vi "Main_18B.vi"() -> ()   [LabVIEW 2024]
uses:
  Utility/Universal Utility/TypeDefs_Utility/Cluster_Row-Column.ctl
  Utility/Universal Utility/TypeDefs_Utility/ENUM_4 Directions U-D-L-R.ctl
  6e548907-4bb0-43d1-b18c-1aae21799752.vi
  855a1de3-eed7-40d2-97cd-9cf78db46282.vi
  <vilib>/Utility/error.llb/Trim Whitespace.vi
  <vilib>/Utility/error.llb/Trim Whitespace One-Sided.vi
panel:
  out "Answer":T1
  out "Started":cluster{"Steps":u64, "Position":T1}[](array[cluster])
  out "sorted array":cluster{"Steps":u64, "Position":T1}[](array[cluster])
  out "Grid":string[][](array[string])
  in  "Puzzle Grid":T1={"R"=70, "C"=70}
  in  "Example Grid":T1={"R"=6, "C"=6}
  in  "Use Puzzle":bool
  out "Steps":u64
  in  "Puzzle":string="60,61\n19,47\n15,43\n15,48\n61,59\n23,51\n29,59\n10,25\n15,50\n26,39\n45,33\n7,29\n57,57\n11,25\n17,38\n3,1\n43,66\n57,55\n19,67\n2,47\n55,49\n13,25\n56,43\n9,2\n7,51\n23,61\n52,65\n11,47\n53,65\n21,47\n3,36\n11,38\n2,3\n1,27\n65,67\n64,63\n39,61\n23,52\n29,67\n69,31\n8,5\n16,69\n9,25\n61,63\n55,53\n7,50\n3,9\n2,41\n12,63\n28,57\n60,65\n55,34\n23,43\n51,68\n68,33\n53,43\n9,52\n21,1\n65,48\n6,27\n57,56\n65,39\n68,69\n67,38\n19,37\n19,63\n16,35\n38,61\n56,39\n24,47\n7,49\n65,59\n11,2\n10,61\n17,64\n60,57\n21,45\n67,59\n65,62\n14,59\n35,65\n37,53\n59,54\n3,19\n59,59\n24,49\n65,35\n5,20\n63,52\n1,51\n7,14\n68,67\n13,65\n8,37\n27,46\n1,12\n28,61\n21,61\n61,54\n41,67\n7,21\n61,58\n69,32\n69,57\n5,33\n1,10\n7,43\n45,57\n25,36\n14,53\n9,43\n27,39\n47,54\n67,41\n9,27\n55,61\n57,63\n65,46\n39,64\n9,33\n63,65\n25,62\n17,48\n8,57\n69,63\n49,35\n47,60\n7,25\n7,41\n59,43\n37,70\n5,28\n18,65\n62,33\n47,67\n19,61\n67,60\n25,44\n69,41\n11,49\n5,37\n12,31\n51,53\n33,63\n23,47\n29,37\n69,55\n23,7\n39,59\n1,0\n39,66\n18,37\n51,57\n10,41\n3,49\n23,39\n59,42\n45,58\n23,56\n67,69\n44,65\n64,69\n4,19\n2,51\n11,43\n1,48\n45,61\n1,29\n32,63\n7,53\n13,27\n52,61\n11,23\n9,63\n5,6\n1,14\n40,69\n19,43\n29,39\n43,69\n53,55\n3,7\n19,62\n27,43\n59,39\n63,57\n41,68\n7,20\n16,45\n26,37\n22,59\n13,47\n13,50\n39,50\n19,29\n51,60\n17,30\n8,61\n9,49\n42,65\n3,31\n56,37\n15,41\n2,31\n5,15\n19,41\n61,32\n1,25\n1,4\n59,67\n6,41\n15,67\n3,35\n61,36\n31,59\n19,3\n65,55\n65,60\n61,55\n57,68\n56,49\n1,19\n3,11\n66,41\n1,15\n66,69\n9,41\n63,39\n2,15\n13,8\n55,32\n19,57\n49,55\n69,40\n67,67\n10,57\n19,51\n2,7\n22,29\n24,41\n5,4\n61,45\n59,63\n11,32\n60,39\n57,35\n24,43\n65,53\n26,69\n21,65\n6,17\n11,34\n67,55\n26,45\n69,43\n30,61\n7,22\n27,47\n7,37\n58,65\n12,41\n9,39\n35,69\n46,63\n13,67\n67,35\n39,69\n15,26\n63,37\n13,45\n43,67\n17,43\n14,61\n57,69\n21,40\n21,56\n69,44\n41,51\n67,43\n37,67\n59,64\n35,59\n0,33\n1,41\n69,56\n31,63\n31,52\n18,57\n13,23\n8,31\n56,53\n7,19\n9,40\n69,66\n9,23\n11,37\n5,29\n22,63\n25,57\n11,46\n1,3\n6,35\n3,2\n8,9\n69,59\n67,49\n53,67\n3,53\n46,67\n49,61\n27,61\n1,33\n54,59\n10,23\n23,41\n6,51\n29,40\n1,37\n14,25\n20,69\n4,35\n15,38\n8,23\n5,19\n23,53\n58,43\n34,63\n63,41\n65,56\n14,43\n21,49\n28,69\n23,57\n57,41\n22,19\n62,35\n11,50\n1,13\n9,20\n28,67\n61,67\n20,43\n58,35\n13,24\n8,53\n3,50\n27,41\n40,67\n0,37\n10,29\n57,39\n31,65\n15,39\n66,51\n10,1\n12,5\n7,44\n3,15\n11,35\n23,38\n58,53\n19,49\n10,65\n39,67\n57,60\n18,67\n33,69\n1,20\n42,63\n37,63\n13,35\n63,55\n11,15\n61,53\n68,59\n51,65\n1,49\n9,46\n19,59\n67,39\n3,45\n50,65\n53,51\n47,61\n65,50\n7,28\n8,35\n21,57\n63,61\n11,33\n3,21\n15,64\n10,15\n25,69\n51,59\n53,39\n7,35\n69,35\n5,10\n3,5\n47,47\n43,65\n37,69\n61,33\n49,56\n25,43\n59,32\n54,55\n51,43\n62,47\n27,69\n10,9\n35,56\n48,67\n57,43\n1,21\n25,41\n5,7\n17,65\n18,39\n61,65\n17,69\n19,45\n55,67\n1,31\n31,57\n17,41\n1,43\n63,43\n44,63\n11,45\n54,69\n55,58\n58,39\n11,36\n4,51\n1,6\n52,67\n16,59\n23,70\n65,61\n59,57\n27,37\n3,16\n56,67\n7,30\n3,47\n3,18\n29,38\n59,36\n69,69\n49,59\n4,25\n43,59\n63,59\n17,47\n0,23\n11,24\n1,1\n37,58\n47,64\n5,48\n5,53\n22,69\n11,29\n61,57\n30,59\n20,59\n11,31\n3,29\n12,43\n15,44\n67,31\n15,36\n43,62\n57,61\n17,39\n67,45\n53,46\n9,3\n18,49\n13,61\n53,62\n66,45\n13,37\n39,65\n11,27\n25,45\n59,69\n21,46\n67,53\n55,70\n17,34\n51,44\n36,61\n63,64\n29,61\n67,37\n61,56\n64,39\n29,65\n42,69\n68,47\n29,36\n17,51\n65,63\n19,32\n69,37\n25,59\n65,33\n13,28\n61,51\n66,53\n38,65\n57,37\n3,38\n11,51\n52,57\n22,41\n65,41\n53,53\n33,56\n27,63\n35,61\n67,44\n69,61\n35,66\n23,45\n3,33\n14,29\n16,65\n61,70\n61,43\n43,57\n7,32\n14,37\n40,63\n61,42\n70,39\n63,40\n53,50\n24,51\n21,39\n2,11\n51,66\n15,62\n62,51\n17,33\n17,29\n51,61\n8,27\n5,45\n53,56\n13,2\n59,52\n61,49\n68,53\n9,51\n58,57\n4,13\n35,63\n21,69\n51,69\n30,63\n12,39\n48,59\n37,68\n45,63\n59,41\n62,67\n5,21\n3,44\n7,42\n19,65\n65,32\n7,17\n64,43\n6,47\n27,60\n1,45\n49,65\n26,63\n1,22\n8,39\n54,33\n7,3\n54,49\n29,63\n65,51\n54,39\n3,37\n9,21\n4,33\n66,57\n7,15\n6,37\n17,46\n58,59\n52,49\n21,37\n1,23\n52,41\n55,64\n3,23\n69,62\n20,41\n2,29\n65,43\n17,67\n29,69\n31,61\n53,42\n51,55\n53,69\n57,67\n7,47\n51,58\n55,57\n63,63\n2,9\n24,59\n17,19\n57,65\n5,2\n0,45\n19,55\n7,23\n9,29\n61,44\n41,61\n25,5\n69,53\n5,47\n51,67\n65,65\n13,40\n2,35\n13,29\n67,48\n9,34\n4,47\n9,53\n21,34\n66,65\n11,41\n2,17\n67,54\n17,59\n11,53\n17,52\n5,25\n4,53\n29,47\n32,61\n15,63\n48,49\n64,55\n25,39\n11,68\n13,64\n65,36\n19,69\n25,48\n24,65\n31,47\n59,65\n55,69\n10,51\n13,46\n27,64\n51,35\n22,49\n69,45\n27,67\n49,68\n65,69\n25,66\n34,61\n68,35\n12,27\n1,39\n59,38\n69,49\n53,61\n49,69\n9,31\n26,59\n51,32\n4,31\n24,57\n64,65\n70,31\n49,57\n63,66\n23,37\n56,41\n35,58\n67,65\n5,35\n57,33\n22,61\n69,46\n17,31\n11,14\n35,64\n64,33\n57,53\n54,61\n37,45\n53,49\n5,39\n8,13\n67,40\n24,37\n67,66\n27,65\n10,43\n0,51\n17,60\n13,31\n7,2\n12,65\n55,59\n33,57\n67,63\n49,46\n21,43\n65,37\n57,59\n21,53\n15,47\n19,36\n59,35\n5,5\n5,31\n61,35\n14,67\n45,68\n6,25\n3,22\n2,43\n50,51\n9,45\n3,26\n20,65\n2,39\n20,47\n61,64\n59,61\n1,42\n3,41\n19,31\n56,57\n43,60\n63,58\n37,65\n58,33\n55,41\n65,49\n53,57\n43,50\n11,48\n5,40\n13,59\n9,57\n26,57\n60,67\n63,67\n6,3\n19,53\n69,67\n59,60\n17,37\n11,26\n28,63\n53,45\n17,27\n17,62\n59,37\n3,28\n49,63\n53,33\n56,61\n6,33\n18,59\n59,68\n41,69\n19,54\n31,37\n62,39\n7,52\n21,52\n27,59\n41,65\n7,7\n11,39\n62,69\n9,47\n16,41\n60,31\n9,59\n11,30\n1,9\n7,1\n21,66\n64,37\n65,57\n69,47\n39,57\n25,47\n5,9\n7,33\n1,17\n69,51\n61,41\n11,16\n6,19\n36,63\n38,57\n55,55\n1,28\n47,69\n4,5\n59,33\n63,35\n62,49\n49,67\n37,61\n5,38\n18,43\n7,0\n54,67\n25,37\n11,66\n67,62\n16,51\n63,69\n5,8\n61,39\n15,29\n68,51\n0,7\n69,64\n21,59\n43,63\n11,7\n63,33\n21,51\n1,26\n49,53\n10,35\n57,34\n70,55\n22,43\n61,38\n3,3\n21,50\n5,27\n23,67\n4,41\n3,17\n20,61\n63,48\n67,51\n66,33\n39,62\n20,53\n68,49\n54,43\n27,5\n25,63\n20,21\n39,63\n55,43\n13,49\n5,23\n8,49\n65,42\n8,25\n4,23\n27,52\n20,37\n53,41\n66,37\n3,25\n18,45\n22,55\n48,65\n9,11\n3,39\n14,31\n65,68\n36,67\n15,66\n55,54\n42,45\n61,69\n3,46\n8,47\n64,53\n69,39\n51,48\n3,13\n2,33\n19,39\n3,27\n33,59\n23,65\n15,30\n23,68\n65,31\n53,59\n55,36\n9,37\n22,25\n19,42\n23,69\n14,49\n17,40\n69,36\n47,65\n55,35\n39,60\n22,37\n60,51\n21,67\n12,47\n9,35\n55,33\n69,65\n68,57\n28,39\n62,55\n57,40\n1,5\n5,44\n65,47\n11,63\n5,1\n54,51\n21,44\n25,61\n61,37\n9,54\n22,65\n25,65\n17,45\n67,42\n67,47\n25,67\n57,66\n23,59\n61,47\n45,66\n62,61\n13,43\n7,16\n45,65\n64,59\n20,31\n17,61\n7,39\n41,63\n27,66\n1,47\n15,65\n21,55\n15,20\n55,52\n18,51\n24,61\n13,41\n62,43\n55,65\n25,68\n67,33\n51,63\n50,43\n23,46\n4,11\n56,63\n5,51\n11,67\n20,57\n5,30\n63,51\n3,24\n14,41\n59,55\n23,49\n15,45\n8,43\n32,65\n66,35\n63,53\n69,60\n15,61\n67,57\n11,13\n61,61\n14,45\n69,42\n25,40\n1,35\n69,33\n63,47\n49,70\n1,11\n61,62\n29,57\n13,63\n33,61\n9,55\n9,58\n62,59\n19,68\n15,49\n69,52\n48,63\n47,56\n17,63\n17,68\n5,49\n20,49\n51,49\n35,9\n5,63\n27,1\n37,39\n37,16\n51,4\n37,8\n63,8\n49,31\n33,13\n59,21\n55,7\n60,49\n36,23\n17,21\n59,17\n19,33\n29,12\n39,35\n13,4\n9,19\n61,7\n45,36\n31,53\n69,0\n25,18\n50,1\n53,15\n60,11\n38,3\n43,25\n13,57\n34,23\n32,23\n63,45\n19,9\n12,61\n39,7\n43,15\n9,13\n47,29\n45,59\n1,7\n47,70\n57,27\n15,56\n37,28\n7,57\n57,10\n40,37\n33,53\n24,5\n25,1\n37,11\n13,14\n51,29\n39,19\n43,17\n49,43\n32,5\n27,19\n35,31\n44,15\n11,9\n49,3\n30,7\n36,27\n41,15\n66,27\n21,9\n43,23\n27,4\n49,39\n39,5\n11,65\n23,9\n56,5\n47,49\n33,28\n48,25\n43,53\n15,53\n48,3\n48,11\n47,2\n29,19\n5,41\n45,30\n49,7\n32,25\n31,69\n65,15\n31,36\n29,17\n23,54\n25,35\n12,53\n69,4\n20,7\n33,27\n63,25\n42,37\n33,12\n53,3\n21,19\n61,21\n45,16\n41,13\n31,30\n53,23\n45,7\n5,55\n31,19\n51,37\n23,1\n27,2\n53,17\n39,51\n40,9\n69,12\n37,37\n13,21\n19,2\n16,3\n35,39\n48,43\n43,49\n29,35\n19,34\n51,19\n15,35\n11,6\n60,23\n21,29\n50,9\n53,11\n53,47\n39,25\n37,54\n28,49\n55,8\n49,19\n21,25\n42,57\n1,61\n1,64\n47,59\n1,65\n59,27\n59,29\n42,27\n55,37\n10,7\n44,1\n15,16\n57,19\n69,17\n54,35\n17,24\n43,51\n13,51\n34,43\n55,63\n69,19\n28,19\n27,21\n31,5\n26,7\n20,63\n51,41\n31,11\n51,45\n45,13\n27,7\n7,68\n23,27\n57,3\n57,25\n25,51\n8,17\n41,28\n32,57\n49,47\n37,34\n26,55\n45,43\n48,29\n51,39\n25,25\n3,57\n56,25\n39,27\n20,9\n27,31\n69,7\n54,47\n69,13\n52,15\n69,3\n62,19\n35,50\n16,17\n27,23\n63,14\n55,16\n61,11\n42,53\n66,5\n31,15\n3,43\n18,9\n17,20\n43,11\n23,21\n62,3\n52,21\n7,5\n33,7\n65,11\n39,46\n61,6\n37,49\n39,49\n31,9\n42,19\n47,33\n31,20\n58,13\n61,8\n24,33\n66,23\n51,40\n35,55\n45,53\n43,55\n35,5\n32,39\n47,21\n41,48\n55,19\n11,59\n45,27\n17,23\n27,24\n23,24\n25,3\n7,59\n35,48\n11,61\n1,62\n64,13\n46,57\n39,0\n6,63\n33,46\n31,13\n33,41\n37,2\n19,5\n48,53\n69,9\n5,54\n33,9\n57,22\n43,7\n15,51\n67,18\n39,44\n41,1\n6,59\n33,43\n57,13\n31,16\n55,5\n31,42\n15,17\n22,15\n42,21\n28,33\n7,66\n37,50\n15,9\n23,8\n21,0\n42,49\n16,27\n29,9\n67,5\n39,17\n11,12\n5,3\n19,18\n59,53\n47,39\n59,9\n45,21\n5,67\n13,11\n15,55\n1,66\n47,28\n49,11\n30,47\n35,32\n41,53\n27,30\n38,39\n44,37\n47,9\n5,13\n31,18\n11,10\n38,7\n37,9\n49,8\n39,31\n29,22\n25,14\n29,53\n12,9\n48,45\n27,55\n13,13\n28,27\n35,30\n38,33\n68,15\n33,37\n69,29\n55,51\n45,67\n65,23\n52,53\n51,25\n15,7\n25,53\n69,14\n44,5\n65,9\n13,15\n51,9\n65,27\n18,27\n51,1\n43,1\n47,7\n51,52\n41,21\n19,4\n23,2\n35,20\n44,55\n37,35\n11,57\n25,55\n40,19\n51,30\n51,5\n9,4\n47,16\n69,21\n25,21\n20,19\n12,59\n10,19\n13,36\n35,42\n43,8\n7,55\n44,45\n37,19\n50,63\n37,13\n55,45\n65,5\n56,7\n57,45\n54,63\n55,0\n35,2\n29,7\n17,13\n30,65\n15,19\n48,19\n7,9\n13,34\n37,1\n31,68\n59,1\n53,35\n41,22\n15,4\n56,23\n11,19\n41,17\n47,25\n19,10\n39,39\n65,1\n21,33\n15,23\n51,20\n40,57\n41,16\n6,69\n45,69\n46,51\n21,21\n45,52\n11,3\n41,57\n36,33\n45,48\n69,15\n67,12\n23,33\n22,13\n59,8\n43,45\n59,13\n29,5\n4,67\n39,55\n38,47\n27,15\n26,19\n70,23\n67,19\n42,55\n30,67\n25,23\n35,3\n25,29\n57,5\n6,55\n39,47\n33,31\n35,68\n47,5\n41,58\n33,65\n29,58\n28,55\n40,55\n67,23\n46,39\n53,13\n51,3\n47,63\n7,56\n43,40\n41,24\n30,5\n26,9\n37,21\n13,56\n31,33\n35,67\n15,33\n7,13\n21,27\n44,21\n46,7\n53,14\n33,55\n15,2\n43,41\n30,45\n59,23\n11,54\n25,19\n35,25\n42,43\n23,63\n37,10\n47,26\n61,1\n15,6\n59,5\n31,2\n21,15\n46,3\n19,35\n3,56\n3,55\n3,63\n47,34\n35,57\n51,31\n41,30\n5,58\n18,7\n32,31\n7,6\n41,5\n48,9\n3,51\n28,17\n33,17\n27,14\n47,27\n41,14\n49,23\n47,19\n24,9\n45,5\n55,9\n9,15\n24,29\n39,3\n39,30\n9,68\n63,10\n54,7\n59,45\n14,7\n36,37\n43,5\n45,18\n65,45\n59,25\n19,27\n67,7\n58,19\n36,11\n13,55\n35,41\n51,33\n33,44\n63,28\n29,41\n12,69\n32,47\n40,25\n46,47\n30,27\n53,19\n23,31\n41,41\n7,67\n68,11\n40,3\n1,63\n22,33\n68,21\n60,19\n7,45\n45,32\n11,5\n49,5\n45,9\n53,16\n65,19\n30,9\n67,29\n55,1\n31,21\n61,12\n63,19\n5,43\n32,41\n41,39\n16,21\n4,63\n62,45\n33,45\n14,17\n17,53\n17,32\n51,7\n56,15\n39,21\n53,2\n43,13\n33,39\n25,49\n50,17\n30,33\n56,27\n41,11\n25,33\n45,40\n47,23\n17,1\n55,15\n59,28\n54,11\n11,17\n57,48\n31,49\n41,55\n15,31\n23,5\n53,27\n35,17\n66,21\n23,19\n33,3\n33,35\n19,15\n69,26\n37,57\n13,22\n38,53\n57,4\n49,1\n41,37\n47,37\n50,37\n67,11\n67,13\n22,7\n29,43\n29,16\n35,29\n41,43\n67,61\n1,69\n30,19\n39,37\n47,43\n65,20\n67,21\n39,15\n51,17\n36,1\n43,31\n42,61\n50,33\n13,0\n21,6\n52,9\n11,1\n19,19\n63,0\n44,3\n26,33\n31,51\n36,25\n49,37\n63,7\n63,49\n39,26\n61,26\n45,45\n13,5\n53,38\n47,45\n18,3\n53,21\n53,31\n21,63\n31,25\n43,27\n15,37\n15,27\n59,24\n25,13\n47,57\n13,20\n13,53\n56,1\n15,25\n33,38\n26,23\n35,36\n43,35\n25,9\n41,3\n46,11\n31,28\n24,3\n25,15\n58,25\n37,48\n45,42\n29,54\n45,25\n17,14\n63,26\n22,27\n40,35\n29,33\n35,23\n38,15\n2,59\n68,27\n19,1\n38,41\n11,55\n23,25\n68,7\n33,40\n31,50\n50,23\n53,5\n2,53\n53,29\n50,49\n23,3\n53,24\n38,27\n65,17\n32,3\n37,31\n30,23\n31,3\n37,3\n19,23\n23,35\n46,5\n24,13\n43,42\n46,45\n34,17\n7,11\n27,57\n26,13\n53,18\n30,55\n69,6\n47,1\n69,1\n49,27\n7,61\n39,13\n39,24\n65,21\n15,5\n27,3\n21,7\n43,6\n59,15\n5,57\n41,32\n3,67\n27,35\n59,30\n45,35\n41,27\n64,21\n39,1\n61,15\n31,27\n14,69\n65,13\n38,5\n59,49\n63,5\n45,11\n60,45\n60,17\n52,35\n31,31\n27,6\n25,26\n51,21\n29,29\n51,38\n68,23\n28,21\n9,62\n47,20\n57,51\n68,19\n15,57\n33,29\n32,59\n1,53\n54,19\n25,20\n9,1\n58,51\n17,6\n37,29\n57,18\n33,68\n42,3\n55,11\n61,14\n56,31\n5,60\n44,27\n20,27\n64,5\n15,1\n37,41\n31,35\n31,45\n67,2\n26,29\n68,17\n42,39\n17,55\n13,33\n31,56\n25,22\n58,1\n37,59\n35,8\n32,53\n35,4\n68,29\n61,2\n48,13\n45,60\n55,21\n47,38\n55,2\n67,8\n17,49\n7,63\n63,1\n7,69\n65,30\n37,22\n51,22\n5,17\n17,11\n37,44\n35,47\n30,13\n33,1\n39,43\n35,16\n13,19\n49,15\n17,18\n36,21\n63,13\n55,29\n65,29\n39,33\n41,45\n34,59\n53,1\n50,7\n17,7\n17,54\n61,5\n21,22\n48,51\n41,25\n48,15\n33,34\n21,5\n46,31\n8,65\n41,4\n47,14\n43,61\n37,7\n1,57\n40,1\n34,51\n61,27\n24,25\n61,23\n17,17\n36,45\n33,67\n69,25\n57,1\n63,3\n14,13\n37,5\n49,49\n37,33\n60,3\n66,25\n29,27\n6,13\n21,31\n59,3\n47,55\n9,17\n34,13\n9,60\n1,68\n47,35\n45,29\n35,37\n60,21\n34,27\n63,21\n67,17\n49,58\n2,55\n63,31\n55,25\n23,6\n15,21\n28,5\n41,59\n43,29\n57,17\n47,13\n25,10\n63,9\n34,37\n52,27\n47,24\n49,29\n11,56\n31,55\n33,26\n53,30\n59,6\n5,61\n37,55\n37,36\n70,9\n42,15\n59,47\n20,25\n3,69\n30,35\n35,11\n59,51\n51,54\n26,1\n55,3\n11,69\n17,3\n51,11\n13,69\n20,29\n53,4\n63,29\n15,69\n67,9\n46,23\n49,22\n41,47\n15,13\n65,24\n9,61\n54,25\n27,49\n5,11\n49,0\n61,3\n15,22\n67,3\n37,17\n29,21\n37,18\n50,3\n28,41\n23,22\n42,1\n55,23\n55,39\n13,9\n21,12\n29,3\n31,39\n38,21\n39,38\n25,27\n66,15\n65,3\n37,51\n45,41\n62,5\n51,27\n27,50\n35,6\n23,11\n47,41\n41,9\n21,17\n45,1\n4,57\n63,11\n45,51\n48,41\n46,49\n35,35\n39,45\n27,53\n46,43\n63,30\n9,18\n28,9\n0,57\n5,62\n52,3\n23,55\n9,9\n51,24\n17,56\n53,63\n35,7\n3,70\n63,12\n2,65\n43,21\n50,27\n20,15\n36,17\n64,3\n57,12\n62,29\n41,31\n33,51\n59,31\n29,13\n37,43\n45,37\n57,31\n34,53\n28,11\n59,19\n49,51\n54,5\n45,44\n45,10\n43,37\n47,22\n9,67\n65,6\n29,0\n19,17\n32,7\n36,13\n57,11\n52,29\n44,23\n29,31\n27,27\n25,0\n69,11\n31,66\n33,47\n21,3\n35,43\n39,9\n49,18\n47,36\n61,17\n29,14\n59,11\n37,25\n29,48\n61,10\n66,3\n57,23\n25,16\n54,27\n15,3\n26,53\n27,13\n67,10\n41,7\n13,10\n50,35\n53,9\n29,49\n53,25\n60,15\n51,51\n70,17\n25,4\n29,25\n63,22\n37,30\n33,20\n37,56\n19,16\n50,55\n33,10\n61,19\n51,13\n58,15\n28,35\n32,33\n61,9\n29,11\n41,49\n31,17\n3,58\n51,12\n35,33\n50,41\n43,9\n35,19\n34,7\n17,9\n69,23\n35,45\n47,51\n31,44\n57,7\n68,3\n30,43\n33,23\n57,49\n41,35\n58,9\n51,23\n17,57\n51,10\n35,51\n38,19\n13,7\n40,39\n67,27\n61,25\n53,7\n40,49\n40,29\n45,34\n51,26\n31,1\n34,9\n3,62\n57,30\n15,15\n43,47\n42,9\n64,1\n13,3\n30,51\n33,19\n9,7\n41,52\n61,4\n40,53\n63,16\n49,21\n44,29\n55,27\n11,22\n34,19\n61,24\n15,32\n19,21\n7,64\n35,49\n13,39\n51,15\n50,13\n17,0\n18,21\n55,22\n45,23\n24,17\n31,7\n27,29\n48,61\n43,43\n57,29\n37,15\n37,47\n33,4\n37,52\n29,45\n31,29\n49,45\n7,8\n5,69\n41,23\n35,15\n38,35\n35,53\n28,43\n43,34\n15,59\n17,5\n31,23\n43,20\n63,24\n27,17\n65,16\n35,21\n47,6\n57,21\n61,29\n63,18\n32,17\n39,41\n23,13\n7,27\n44,51\n1,55\n33,5\n3,65\n7,65\n47,31\n54,21\n17,35\n27,33\n65,10\n53,10\n53,37\n49,9\n13,58\n48,31\n19,11\n45,8\n25,17\n63,23\n23,23\n33,25\n3,59\n10,13\n22,17\n25,54\n39,11\n33,33\n44,11\n22,11\n33,21\n45,26\n26,27\n34,1\n27,51\n52,37\n44,57\n63,15\n18,11\n46,27\n46,13\n26,49\n3,61\n29,32\n67,1\n47,15\n45,31\n12,17\n50,31\n59,7\n23,29\n28,45\n55,17\n27,45\n49,25\n24,31\n43,19\n16,57\n65,7\n19,7\n38,13\n34,31\n47,11\n69,27\n4,65\n42,11\n42,17\n32,51\n4,15\n45,49\n27,11\n25,32\n33,14\n9,69\n43,33\n39,29\n17,15\n65,25\n69,5\n47,17\n52,45\n11,11\n49,13\n57,9\n41,46\n58,47\n8,69\n13,52\n31,41\n45,39\n9,5\n41,29\n56,13\n43,32\n58,3\n46,19\n6,11\n30,29\n20,3\n45,3\n17,28\n18,25\n48,39\n60,47\n61,13\n19,25\n25,31\n22,31\n44,13\n29,23\n37,23\n38,11\n5,46\n40,17\n1,67\n21,13\n40,43\n49,41\n33,15\n27,25\n30,3\n21,23\n12,19\n45,19\n47,3\n34,35\n1,59\n58,21\n69,28\n48,35\n29,26\n63,17\n8,11\n67,30\n20,23\n54,45\n22,3\n43,39\n18,15\n24,35\n55,13\n33,11\n29,15\n23,15\n39,14\n56,45\n38,43\n15,12\n16,11\n35,40\n45,55\n52,19\n13,1\n51,47\n56,11\n44,47\n41,19\n5,59\n62,21\n29,8\n29,24\n41,12\n40,41\n31,67\n65,8\n47,53\n49,17\n39,8\n28,29\n25,11\n49,6\n45,54\n49,33\n25,7\n23,17\n45,17\n32,11\n45,47\n58,45\n65,18\n35,13\n29,51\n55,28\n35,46\n59,16\n34,25\n19,13\n13,17\n67,15\n1,60\n5,65\n27,9\n23,20\n43,3\n29,55\n42,31\n57,15\n17,12\n7,31\n41,6\n20,13\n39,53\n63,27\n53,6\n15,8\n33,49\n39,23\n21,11\n35,1\n61,31\n57,28\n55,47\n31,43\n35,54\n40,5\n26,11\n21,35\n43,24\n50,15\n36,41\n18,29\n45,15\n57,47\n11,21\n3,68\n17,25\n21,41\n37,27\n60,27\n67,25\n42,35\n9,65\n33,48\n33,70\n64,27\n56,19\n35,27\n15,11\n41,33\n55,31\n29,1\n30,16\n57,26\n52,16\n36,7\n41,2\n36,29\n6,22\n68,61\n27,16\n56,9\n60,54\n70,37\n66,49\n61,40\n12,55\n0,42\n44,41\n40,48\n64,52\n56,6\n12,8\n63,50\n26,28\n17,26\n47,12\n21,18\n66,48\n66,4\n52,22\n54,46\n47,42\n28,60\n60,41\n64,42\n40,51\n24,18\n0,59\n63,2\n3,32\n31,64\n6,24\n58,48\n42,60\n60,33\n42,8\n5,24\n46,69\n48,37\n58,64\n24,24\n20,39\n0,70\n58,14\n42,20\n54,3\n70,56\n24,62\n2,16\n2,10\n50,47\n38,37\n26,21\n22,58\n59,10\n0,50\n61,28\n51,18\n53,34\n30,31\n0,5\n18,23\n22,40\n60,10\n49,10\n19,30\n52,7\n32,9\n57,58\n20,16\n26,42\n50,19\n8,20\n16,58\n66,56\n21,10\n45,6\n64,15\n22,4\n63,42\n5,0\n42,44\n6,23\n52,10\n16,38\n55,48\n16,40\n62,14\n2,64\n52,63\n22,42\n65,2\n56,65\n47,0\n24,15\n62,13\n11,64\n68,30\n29,20\n0,58\n54,64\n12,7\n43,10\n50,60\n37,38\n0,56\n27,10\n66,50\n54,17\n20,6\n1,56\n16,0\n33,18\n49,34\n62,25\n39,12\n58,8\n32,64\n36,0\n56,2\n66,42\n35,12\n28,0\n26,20\n10,5\n63,60\n39,28\n6,12\n56,52\n62,56\n44,67\n36,30\n41,26\n70,34\n59,26\n6,32\n60,0\n40,54\n12,30\n50,6\n16,37\n46,42\n70,46\n20,70\n46,34\n4,66\n25,42\n36,60\n60,5\n10,18\n68,6\n47,58\n38,38\n40,0\n24,20\n25,12\n5,50\n48,22\n12,37\n18,36\n70,16\n36,59\n14,60\n39,18\n58,17\n10,47\n4,44\n10,40\n30,60\n42,24\n8,18\n51,64\n12,34\n14,24\n40,52\n46,25\n4,12\n55,14\n60,34\n1,16\n55,18\n41,10\n66,64\n54,37\n38,26\n50,10\n67,70\n69,50\n43,36\n56,40\n6,8\n18,41\n46,60\n36,58\n13,44\n53,58\n10,2\n10,60\n46,55\n70,66\n15,14\n54,22\n62,23\n57,32\n42,6\n9,24\n31,8\n57,38\n46,14\n60,42\n1,44\n36,5\n49,28\n4,50\n63,44\n46,15\n57,62\n2,44\n70,8\n56,17\n59,12\n68,66\n68,64\n36,34\n30,17\n60,37\n54,34\n0,49\n62,17\n37,26\n64,2\n14,22\n10,12\n28,1\n50,0\n0,32\n0,65\n43,38\n67,56\n33,60\n18,34\n60,12\n59,58\n36,20\n49,40\n42,36\n70,2\n2,27\n7,4\n19,70\n64,32\n44,36\n56,48\n14,8\n14,35\n54,15\n68,2\n16,12\n36,28\n23,18\n18,12\n45,4\n12,33\n12,3\n36,6\n37,32\n64,8\n66,18\n64,14\n16,53\n69,38\n44,7\n58,68\n22,36\n52,36\n70,6\n0,66\n7,48\n59,0\n37,20\n69,2\n17,22\n14,52\n61,66\n46,33\n46,28\n35,18\n38,50\n24,42\n42,14\n43,0\n64,16\n7,70\n54,54\n1,58\n70,62\n0,69\n4,14\n11,44\n43,44\n61,52\n0,6\n45,24\n60,59\n20,40\n26,43\n70,52\n30,37\n2,13\n41,38\n58,30\n51,36\n42,29\n68,39\n26,54\n52,43\n20,62\n65,12\n68,40\n1,46\n24,32\n10,44\n12,56\n58,52\n37,60\n68,55\n62,41\n30,26\n40,38\n15,40\n3,10\n38,24\n40,50\n46,24\n24,12\n36,15\n32,35\n20,8\n70,36\n50,28\n52,38\n31,34\n64,26\n28,6\n52,60\n10,20\n66,11\n52,0\n64,46\n26,32\n4,48\n36,68\n11,70\n34,20\n42,32\n32,21\n54,52\n34,0\n68,9\n40,10\n28,42\n26,24\n58,61\n2,25\n28,36\n66,44\n28,38\n66,0\n40,20\n0,68\n57,46\n12,58\n19,26\n14,2\n49,52\n3,48\n65,44\n60,63\n34,64\n42,30\n6,43\n68,50\n48,24\n14,5\n16,64\n52,2\n13,16\n6,49\n4,17\n16,22\n16,2\n56,66\n44,9\n60,25\n66,10\n3,66\n30,20\n31,6\n8,16\n22,30\n52,39\n46,1\n70,32\n28,10\n23,62\n37,24\n12,15\n45,0\n32,32\n22,26\n49,44\n32,24\n10,21\n50,26\n56,22\n22,5\n30,34\n64,31\n5,64\n52,46\n62,54\n51,56\n30,66\n50,50\n43,14\n28,44\n14,15\n16,13\n8,21\n10,11\n28,8\n42,33\n21,20\n45,22\n32,6\n2,57\n32,19\n60,28\n70,63\n33,6\n34,14\n6,67\n39,56\n41,8\n55,10\n50,22\n8,22\n10,10\n9,0\n46,62\n49,32\n14,33\n29,28\n56,3\n44,2\n51,16\n31,24\n43,2\n20,38\n52,20\n24,7\n12,4\n22,10\n28,53\n44,38\n43,56\n32,55\n56,58\n26,38\n61,60\n38,20\n40,27\n12,26\n53,28\n26,8\n47,32\n52,40\n38,9\n20,5\n9,8\n48,7\n58,11\n46,61\n38,18\n57,24\n14,39\n39,58\n30,2\n70,35\n67,28\n30,38\n62,28\n30,36\n3,12\n38,28\n36,26\n70,10\n13,38\n36,52\n46,35\n9,14\n56,20\n55,4\n35,10\n42,10\n28,16\n64,61\n61,20\n50,8\n55,12\n4,60\n65,64\n26,15\n21,28\n70,64\n26,30\n28,14\n58,62\n62,52\n16,54\n20,44\n1,54\n34,12\n28,22\n2,21\n28,20\n70,27\n23,64\n2,62\n33,62\n34,3\n22,22\n44,30\n56,29\n70,7\n25,24\n65,0\n14,62\n54,48\n47,30\n10,8\n8,62\n62,31\n1,38\n45,12\n67,16\n36,35\n34,36\n8,19\n47,50\n8,68\n13,62\n28,26\n18,26\n12,50\n64,28\n55,46\n46,22\n64,22\n58,28\n7,54\n34,18\n0,62\n18,38\n4,4\n3,4\n40,2\n58,22\n19,14\n24,56\n13,26\n38,67\n22,1\n54,50\n61,46\n14,50\n40,59\n40,60\n10,31\n68,46\n30,1\n40,68\n34,55\n2,6\n18,55\n52,62\n61,34\n36,47\n4,27\n42,67\n41,34\n4,69\n16,7\n8,12\n45,20\n5,14\n18,69\n19,24\n66,39\n43,12\n55,20\n66,60\n3,34\n56,35\n28,15\n24,8\n12,42\n20,2\n30,57\n22,18\n50,29\n20,22\n15,10\n4,32\n31,40\n20,26\n18,50\n69,22\n48,55\n40,47\n48,16\n40,58\n39,34\n44,35\n58,58\n32,46\n6,29\n45,28\n56,4\n14,32\n2,48\n50,58\n41,36\n59,66\n23,4\n28,23\n66,52\n19,48\n8,36\n2,20\n48,56\n8,0\n25,30\n18,30\n62,62\n61,18\n10,53\n52,33\n68,70\n26,40\n27,62\n57,36\n10,6\n27,12\n45,56\n10,4\n46,21\n55,66\n20,52\n48,38\n49,12\n70,14\n64,20\n70,49\n30,25\n44,34\n27,26\n27,68\n4,46\n6,15\n43,28\n50,66\n38,22\n12,66\n38,62\n30,70\n18,4\n30,50\n19,40\n52,48\n60,44\n24,45\n16,70\n19,6\n56,8\n29,64\n5,18\n0,17\n48,12\n65,26\n70,20\n56,38\n62,16\n66,63\n60,29\n14,12\n54,32\n10,55\n6,7\n48,27\n60,9\n28,7\n66,24\n9,6\n0,20\n12,40\n35,62\n48,70\n64,54\n22,56\n53,12\n35,0\n28,13\n14,46\n8,38\n20,18\n12,25\n49,14\n14,63\n54,36\n0,2\n62,50\n50,45\n43,64\n14,28\n50,64\n52,14\n44,48\n34,28\n43,16\n32,18\n53,52\n4,24\n42,70\n16,4\n44,66\n4,0\n67,46\n24,27\n4,45\n70,4\n36,70\n33,0\n42,62\n38,17\n24,69\n19,50\n56,64\n7,60\n2,66\n67,68\n60,18\n48,34\n62,63\n31,14\n0,1\n53,32\n13,54\n16,6\n66,17\n52,17\n49,60\n68,1\n64,70\n54,1\n18,14\n53,54\n38,56\n44,64\n7,38\n23,10\n58,38\n45,62\n36,22\n33,66\n65,34\n20,46\n19,28\n2,2\n44,22\n8,52\n2,63\n16,14\n58,44\n65,38\n16,20\n40,15\n17,50\n4,2\n7,62\n62,11\n18,19\n69,48\n44,0\n44,17\n32,8\n68,44\n18,32\n22,24\n32,36\n66,54\n46,54\n40,8\n20,66\n46,46\n50,38\n52,23\n34,58\n10,67\n55,24\n30,53\n2,22\n28,52\n14,4\n43,4\n30,41\n24,11\n8,48\n52,32\n14,1\n20,48\n47,48\n0,29\n4,16\n2,37\n13,48\n68,42\n32,56\n66,40\n44,24\n66,46\n2,54\n2,8\n57,70\n60,66\n54,26\n45,46\n62,20\n37,40\n25,46\n20,34\n29,34\n0,30\n43,70\n38,58\n28,40\n3,30\n7,12\n34,2\n4,21\n13,68\n36,51\n34,42\n17,10\n43,46\n26,36\n30,54\n44,8\n58,31\n16,16\n8,45\n18,56\n48,18\n12,44\n0,52\n18,44\n4,1\n56,60\n7,46\n26,16\n64,25\n58,69\n62,40\n28,64\n22,14\n38,4\n27,38\n19,12\n64,60\n55,68\n54,57\n8,7\n8,46\n25,56\n5,16\n31,62\n68,45\n0,8\n22,8\n44,25\n21,26\n9,56\n48,54\n22,47\n66,47\n50,5\n33,16\n23,14\n38,40\n57,50\n31,38\n0,55\n36,31\n66,19\n24,39\n23,34\n47,4\n3,20\n54,29\n62,1\n55,30\n57,64\n64,29\n16,29\n22,21\n34,45\n38,14\n4,22\n58,29\n16,47\n52,44\n8,64\n22,12\n34,67\n9,10\n12,28\n36,65\n22,53\n67,22\n40,28\n30,44\n50,48\n22,35\n0,48\n6,14\n4,55\n23,30\n24,58\n33,32\n57,8\n39,10\n64,50\n23,12\n40,56\n4,29\n49,2\n36,16\n19,22\n0,46\n32,28\n16,56\n36,69\n21,14\n38,23\n48,21\n69,58\n16,55\n10,66\n56,55\n15,58\n18,17\n10,14\n9,32\n0,21\n0,26\n2,40\n48,2\n30,0\n10,70\n50,34\n66,61\n14,27\n0,10\n18,8\n28,31\n22,32\n12,24\n51,50\n17,2\n8,10\n29,46\n62,0\n9,64\n54,60\n16,68\n38,8\n36,57\n23,16\n22,62\n70,3\n26,70"
  in  "Example":string="5,4\n4,2\n4,5\n3,0\n2,1\n6,3\n2,4\n1,5\n0,6\n3,3\n2,6\n5,1\n1,2\n5,5\n2,5\n6,5\n1,4\n0,4\n6,4\n1,1\n6,1\n1,0\n0,5\n1,6\n2,0"
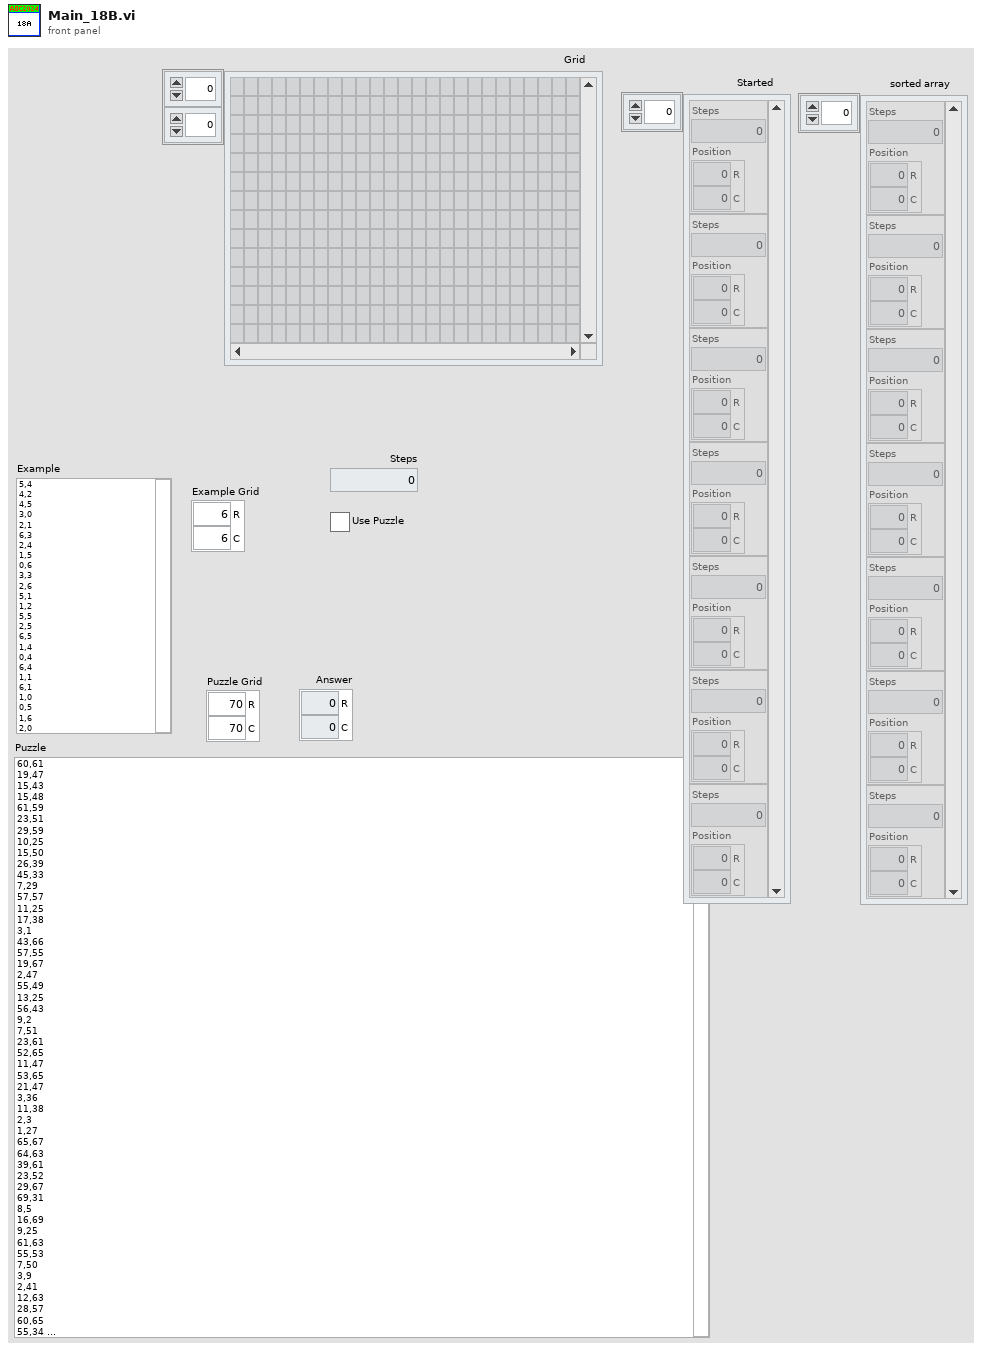
[diagram p1: front panel]
types:
  T1 = typedef "Cluster_Row-Column.ctl" = cluster{"R":i32, "C":i32}
  T2 = typedef "ENUM_4 Directions U-D-L-R.ctl" = enum16{"Up;-1,0", "Right;0,1", "Down;1,0", "Left;0,-1"}
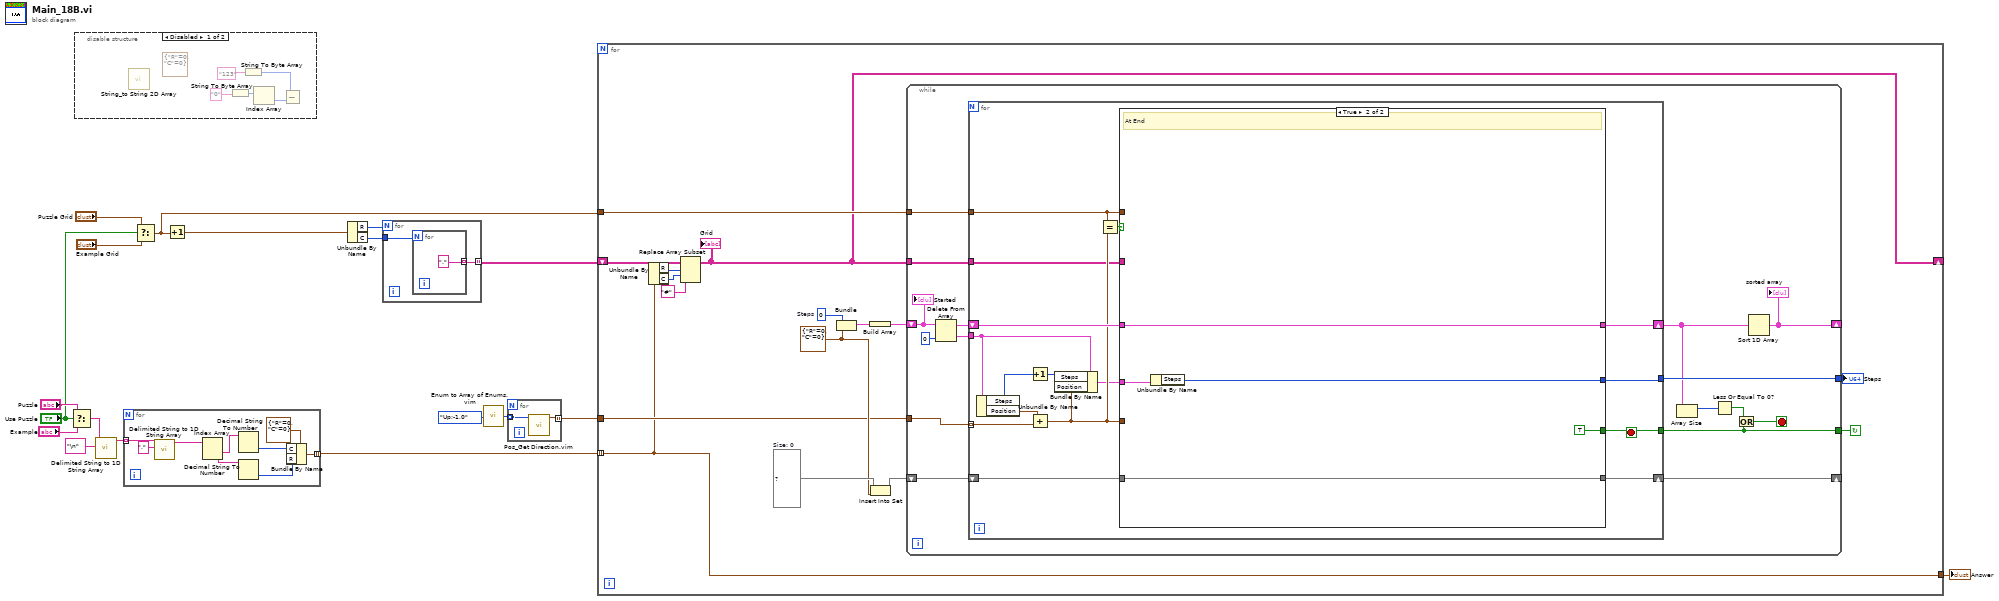
[diagram p0: block diagram]
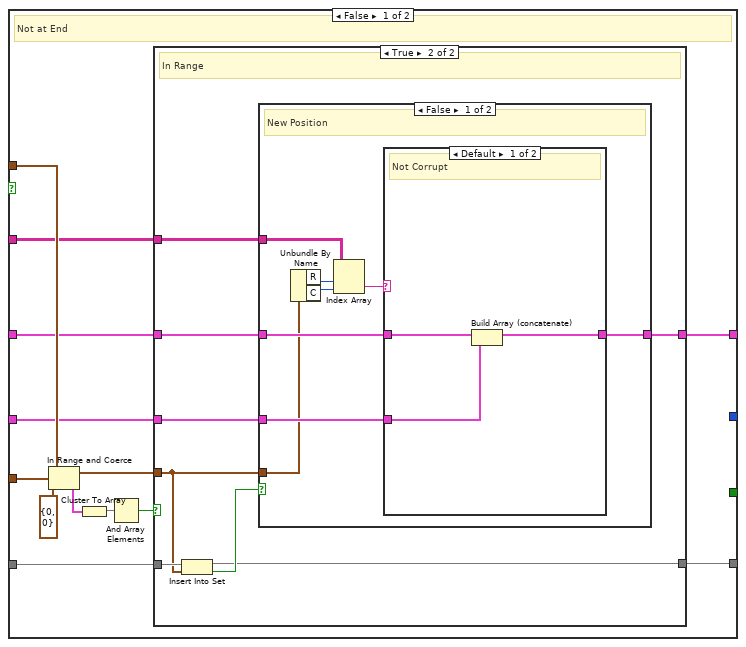
[diagram p2: hidden frame]
diagram:
  n1 = Select(t="Puzzle", s="Use Puzzle", f="Example") -> (s? t:f=w15:string)
  n2 = disable-structure shown="Disabled" {
    frame Disabled {
      (unwired) T1 {"R"=0, "C"=0} ("Position")
      n3 = call "String_to String 2D Array.vi"() -> ()  [unwired: 11 in, 1 out]
      n4 = String To Byte Array(string="0") -> (unsigned byte array=w21:u8[])
      n5 = String To Byte Array(string="123") -> (unsigned byte array=w19:u8[])
      n6 = Index Array(array=w21) -> (element=w20:u8)  [unwired: 1 in]
      n7 = Subtract(x=w19, y=w20) -> ()  [unwired: 1 out]
    }
    frame Enabled {
    }
  }
  n8 = call <vilib>:"Delimited String to 1D String Array.vi"("delimiter"="\n" ("delimiter (Tab)"), "delimited string"=w15) -> ("string array"=w17:string[])  [unwired: 9 in]
  n9 = for {
    tunnel: w17 -> [w32] mode=indexing
    tunnel: [w24] -> w5 mode=indexing
    n10 = call <vilib>:"Delimited String to 1D String Array.vi"("delimiter"=",", "delimited string"=w32) -> ("string array"=w30:string[])  [unwired: 9 in]
    n11 = Index Array(array=w30) -> (element #1=w29:string, element #2=w28:string)  [unwired: 2 in]
    n12 = Decimal String To Number(string=w29) -> (number=w26:i32)  [unwired: 2 in, 1 out]
    n13 = Decimal String To Number(string=w28) -> (number=w25:i32)  [unwired: 2 in, 1 out]
    n14 = Bundle By Name(cluster=T1 {"R"=0, "C"=0} ("Position"), "C"=w26, "R"=w25) -> (w24:T1)
  }
  n15 = Select(t="Puzzle Grid", s="Use Puzzle", f="Example Grid") -> (s? t:f=w6:T1)
  n16 = Increment(x=w6) -> (x+1=w7:T1)
  n17 = Unbundle By Name(w7) -> ("R"=w10:i32, "C"=w9:i32)
  n18 = for {
    N: w10 -> [_]
    tunnel: w9 -> [w34]
    tunnel: [w33] -> w8 mode=indexing
    n19 = for {
      N: w34 -> [_]
      tunnel: ["."] -> w33 mode=indexing
    }
  }
  n20 = call "Enum to Array of Enums.vim"("enum"=ENUM_4_Directions_U-D-L-R."Up;-1,0" ("Direction")) -> ("array of enums"=w4:T2[])
  n21 = for {
    tunnel: w4 -> [w37] mode=indexing
    tunnel: [w36] -> w2 mode=indexing
    n22 = call "Pos_Get Direction.vim"("Direction"=w37) -> ("Position"=w36:T1)  [unwired: 10 in]
  }
  n23 = for {
    tunnel: w6 -> [w49]
    tunnel: w5 -> [w40] mode=indexing
    tunnel: w2 -> [w41]
    tunnel: [w40] -> w1
    shift-right: [w38] -> _
    shift-left: w8 -> [w53]
    stop <- w39 continue-if-true
    w47 = set{T1} {}  # Size: 0
    w52 = u64 0  # Steps
    w45 = T1 {"R"=0, "C"=0} ("Position")
    n24 = Unbundle By Name(w40) -> ("R"=w44:i32, "C"=w43:i32)
    n25 = Replace Array Subset(array=w53, new element="#" ("new element/subarray"), index (row)=w44, index (col)=w43) -> (w38:string[][])
    "Grid" <- w38
    n26 = Bundle("Steps"=w52, "Position"=w45) -> (w51:cluster{"Steps":u64, "Position":T1})  [unwired: 1 in]
    n27 = Build Array(w51) -> (w50:cluster{"Steps":u64, "Position":T1}[])
    n28 = Insert Into Set(10:w45, 11:w47) -> (3:w46:set{T1})  [unwired: 1 out]
    n29 = while {
      tunnel: w38 -> [w64]
      shift-right: [w60] -> _
      shift-left: w50 -> [w69]
      tunnel: w49 -> [w65]
      tunnel: [w63] -> w48
      shift-right: [w61] -> _
      shift-left: w46 -> [w62]
      tunnel: w41 -> [w56]
      tunnel: [w54] -> w39
      stop <- w57 stop-if-true
      n30 = Delete From Array(array=w69, index=0) -> (deleted portion=w67:cluster{"Steps":u64, "Position":T1}, array with subset deleted=w66:cluster{"Steps":u64, "Position":T1}[])  [unwired: 1 in]
      n31 = for {
        tunnel: w56 -> [w85] mode=indexing
        tunnel: w67 -> [w80]
        shift-right: [w74] -> w59
        shift-left: w66 -> [w81]
        tunnel: w65 -> [w83]
        tunnel: w64 -> [w75]
        tunnel: [w73] -> w63
        tunnel: [w72] -> w54
        shift-right: [w70] -> w61
        shift-left: w62 -> [w71]
        stop <- w72 stop-if-true
        n32 = Unbundle By Name(w80) -> ("Steps"=w79:u64, "Position"=w84:T1)
        n33 = Increment(x=w79) -> (x+1=w78:u64)
        n34 = Add(x=w84, y=w85) -> (x+y=w77:T1)
        n35 = Bundle By Name(cluster=w80, "Steps"=w78, "Position"=w77) -> (w76:cluster{"Steps":u64, "Position":T1})
        n36 = Equal?(x=w83, y=w77) -> (x = y?=w82:bool)
        n37 = case shown="True" w82 {
          tunnel: w77 -> [w98 _]
          tunnel: w83 -> [w96 _]
          tunnel: w81 -> [w92 w123]
          tunnel: w76 -> [w93 w125]
          tunnel: w75 -> [w95 _]
          tunnel: [w91 w123] -> w74
          tunnel: [_ TRUE] -> w72
          tunnel: [_ w124] -> w73
          tunnel: w71 -> [w90 w122]
          tunnel: [w89 w122] -> w70
          frame False {
            # "Not at End"
            n38 = In Range and Coerce(upper limit=w96, x=w98, lower limit=T1 {"R"=0, "C"=0}) -> (coerced(x)=w94:T1, In Range?=w88:cluster{"R":bool, "C":bool})
            n39 = Cluster To Array(cluster=w88) -> (array=w87:bool[])
            n40 = And Array Elements(Boolean array=w87) -> (logical AND=w86:bool)
            n41 = case shown="True" w86 {
              tunnel: w95 -> [_ w108]
              tunnel: w94 -> [_ w103]
              tunnel: w93 -> [_ w107]
              tunnel: w92 -> [w100 w106]
              tunnel: [w100 w105] -> w91
              tunnel: w90 -> [w99 w104]
              tunnel: [w99 w101] -> w89
              frame False {
                # "Out of Range"
              }
              frame True {
                # "In Range"
                n42 = Insert Into Set(10:w103, 11:w104) -> (2:w102:bool, 3:w101:set{T1})
                n43 = case shown="False" w102 {
                  tunnel: w108 -> [w116 _]
                  tunnel: w107 -> [w112 _]
                  tunnel: w106 -> [w111 w121]
                  tunnel: [w110 w121] -> w105
                  tunnel: w103 -> [w109 _]
                  frame False {
                    # "New Position"
                    n44 = Unbundle By Name(w109) -> ("R"=w115:i32, "C"=w114:i32)
                    n45 = Index Array(array=w116, index (row)=w115, index (col)=w114) -> (element=w113:string)
                    n46 = case shown="Default" w113 {
                      tunnel: w112 -> [w117 _]
                      tunnel: w111 -> [w119 w120]
                      tunnel: [w118 w120] -> w110
                      frame Default {
                        # "Not Corrupt"
                        n47 = Build Array (concatenate)(w119, w117) -> (w118:cluster{"Steps":u64, "Position":T1}[])
                      }
                      frame "#" {
                        # "Corrupt"
                      }
                    }
                  }
                  frame True {
                    # "Already Evaluated"
                  }
                }
              }
            }
          }
          frame True {
            # "At End"
            n48 = Unbundle By Name(w125) -> ("Steps"=w124:u64)
          }
        }
      }
      n49 = Array Size(array=w59) -> (size(s)=w58:i32)
      n50 = Less Or Equal To 0?(x=w58) -> (x <= 0?=w55:bool)
      n51 = Or(x=w55, y=w54) -> (x .or. y?=w57:bool)
      n52 = Sort 1D Array(array=w59) -> (sorted array=w60:cluster{"Steps":u64, "Position":T1}[])
      "sorted array" <- w60
      "Started" <- w69
    }
    "Steps" <- w48
  }
  "Answer" <- w1
